vi "TDC_setTimestampBufferSize.vi"(8 "Error In":errorcluster, 11 "Buffer Size":i32 min=1 max=1000000) -> (0 "Error Out":errorcluster)   [LabVIEW 2011]
uses:
  dist/userlib/lib/tdcbase.dll
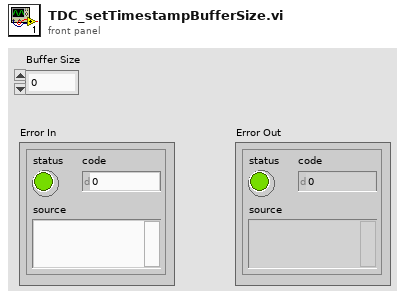
[diagram p1: front panel]
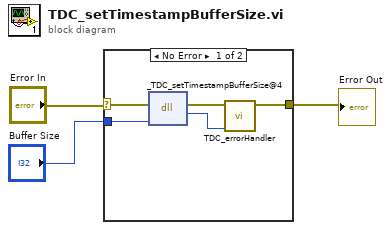
[diagram p0: block diagram]
diagram:
  n1 = case shown="No Error" "Error In" {
    selector: "Error In" -> [w7 w9]
    tunnel: [w4 w9] -> w3
    tunnel: "Buffer Size" -> [w8 _]
    frame No Error {
      n2 = dll-call lib="C:/nh/projekt/spmctrl/dist/userlib/lib/tdcbase.dll" fn="_TDC_setTimestampBufferSize@4"(error in=w7, "bufferSize"=w8) -> (error out=w6:errorcluster, "return type"=w5:i32)  [unwired: 3 in, 1 out]
      n3 = call "TDC_errorHandler.vi"("quTAU Return Code"=w5, "Error In"=w6) -> ("Error Out"=w4:errorcluster)  [unwired: 9 in]
    }
    frame Error {
    }
  }
  "Error Out" <- w3
